vi "Base File Path.vi"() -> (3 "Paths Out":T1)   [LabVIEW 2016]
uses:
  File Paths.ctl
panel:
  in  "Paths":T1
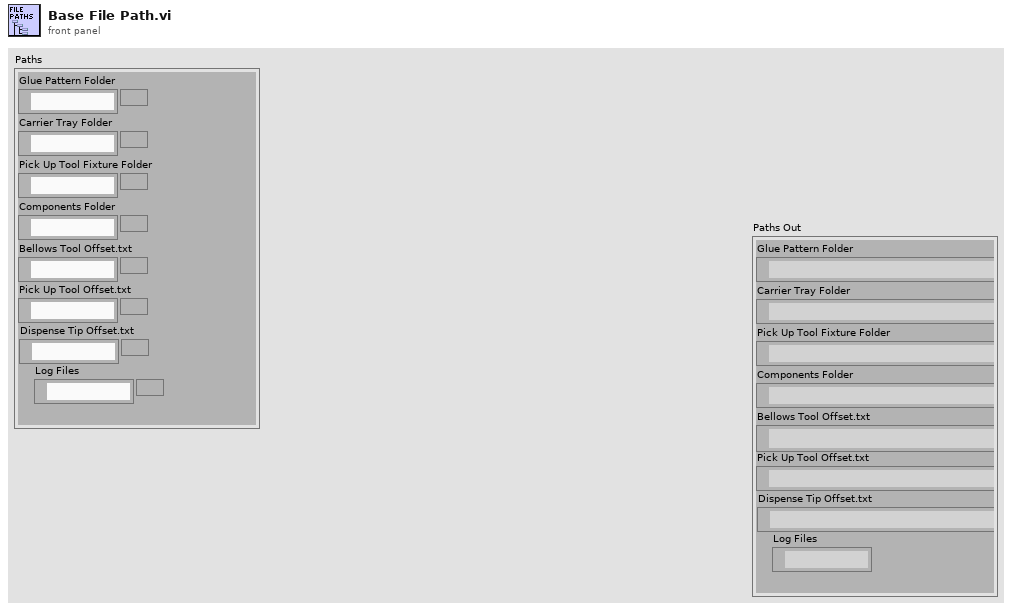
[diagram p1: front panel]
types:
  T1 = typedef "File Paths.ctl" = cluster{"Glue Pattern Folder":path, "Carrier Tray Folder":path, "Pick Up Tool Fixture Folder":path, "Components Folder":path, "Bellows Tool Offset.txt":path, "Pick Up Tool Offset.txt":path, "Dispense Tip Offset.txt":path, "Log Files":path}
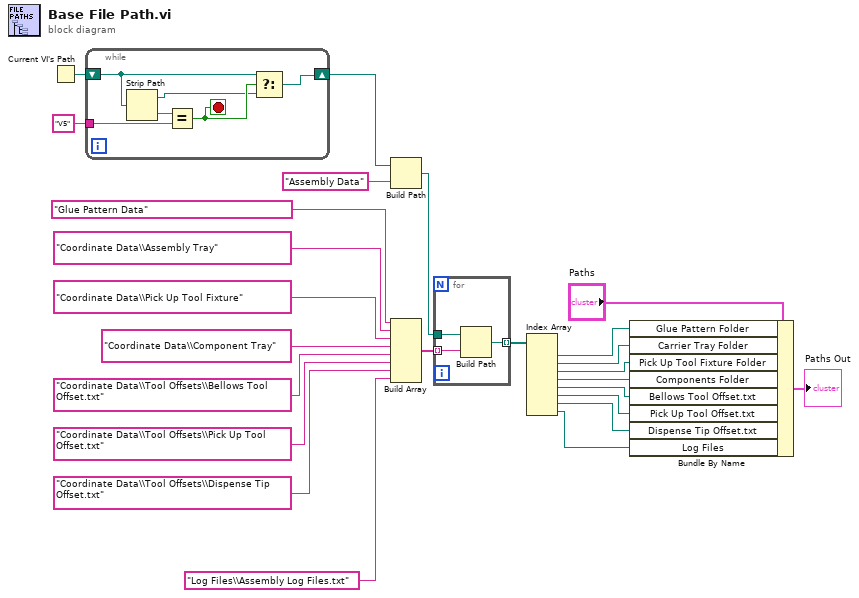
[diagram p0: block diagram]
diagram:
  n1 = Current VI's Path() -> (path=w25:path)
  n2 = while {
    shift-right: [w27] -> w21
    shift-left: w25 -> [w29]
    tunnel: "V5" -> [w26]
    stop <- w30 stop-if-true
    n3 = Strip Path(path=w29) -> (stripped path=w28:path, name=w31:string)
    n4 = Equal?(x=w31, y=w26) -> (x = y?=w30:bool)
    n5 = Select(t=w29, s=w30, f=w28) -> (s? t:f=w27:path)
  }
  n6 = Build Path(base path=w21, name or relative path="Assembly Data") -> (appended path=w19:path)
  n7 = Build Array("Glue Pattern Data", "Coordinate Data\\Assembly Tray", "Coordinate Data\\Pick Up Tool Fixture", "Coordinate Data\\Component Tray" ("element"), "Coordinate Data\\Tool Offsets\\Bellows Tool Offset.txt", "Coordinate Data\\Tool Offsets\\Pick Up Tool Offset.txt", "Coordinate Data\\Tool Offsets\\Dispense Tip Offset.txt", "Log Files\\Assembly Log Files.txt") -> (w11:string[])
  n8 = for {
    tunnel: w19 -> [w34]
    tunnel: [w33] -> w23 mode=indexing
    tunnel: w11 -> [w32] mode=indexing
    n9 = Build Path(base path=w34, name or relative path=w32) -> (appended path=w33:path)
  }
  n10 = Index Array(array=w23) -> (element #1=w10:path, element #2=w9:path, element #3=w8:path, element #4=w7:path, element #5=w6:path, element #6=w5:path, element #7=w4:path, element #8=w1:path)  [unwired: 8 in]
  n11 = Bundle By Name(cluster="Paths", "Glue Pattern Folder"=w10, "Carrier Tray Folder"=w9, "Pick Up Tool Fixture Folder"=w8, "Components Folder"=w7, "Bellows Tool Offset.txt"=w6, "Pick Up Tool Offset.txt"=w5, "Dispense Tip Offset.txt"=w4, "Log Files"=w1) -> (→"Paths Out":T1)
